vi "Tosca-Monitor Trial-State.vi"(0 "DI":bool[](array[boolean]), 7 "Trial/State In":bool[](array[boolean])) -> (8 "Trial/State out":bool[](array[boolean]), 10 "Any change":bool, 13 "State change?":bool)   [LabVIEW 2020]
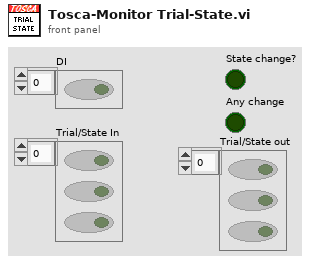
[diagram p1: front panel]
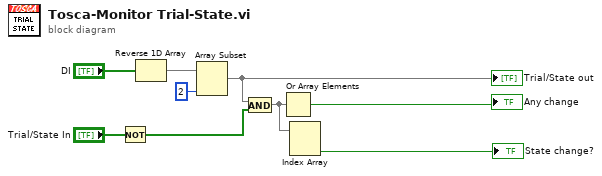
[diagram p0: block diagram]
diagram:
  n1 = Not(x="Trial/State In") -> (.not. x?=w4:bool[])
  n2 = Reverse 1D Array(array="DI") -> (reversed array=w8:bool[])
  n3 = Array Subset(array=w8, length=2) -> (w6:bool[])  [unwired: 1 in]
  "Trial/State out" <- w6
  n4 = And(x=w6, y=w4) -> (x .and. y?=w2:bool[])
  n5 = Or Array Elements(Boolean array=w2) -> (logical OR=→"Any change":bool)
  n6 = Index Array(array=w2) -> (element #2=→"State change?":bool)  [unwired: 2 in, 1 out]
